vi "SetToRandomPosition.vi"(8 "error in (no error)":errorcluster, 10 "BlockedSpots":T1[](array[typedef]), 11 "SnakeSwitch in":refnum<class "SnakeSwitch.lvclass">) -> (0 "error out":errorcluster, 3 "SnakeSwitch out":refnum<class "SnakeSwitch.lvclass">)   [LabVIEW 2019, in "RT_Game.lvlib" / "SnakeSwitch.lvclass"]
uses:
  SnakeSwitch.lvclass
  C:/Users/FreshBob/Dropbox/VIs/myRIO_GameConsole/RT/RT_Game/GameObject/GameObject.lvclass
  Game/Coordinate.ctl
  GameObject/GameObject.lvclass/GameObject.ctl
  GameObject/Write position.vi
  Game/Game.lvclass
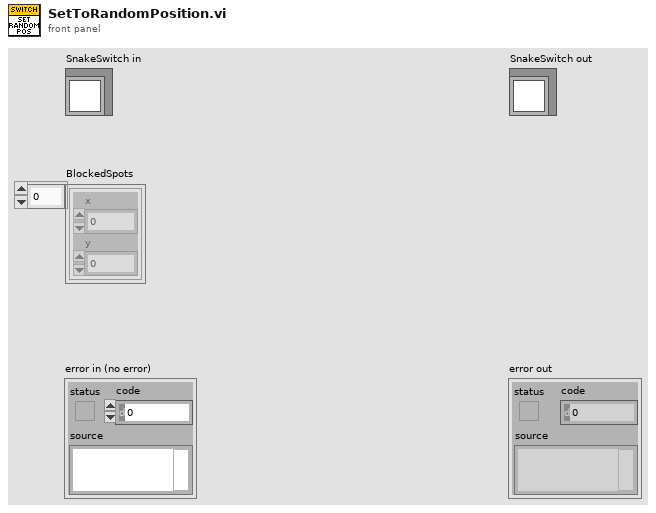
[diagram p1: front panel]
types:
  T1 = typedef "RT_Game.lvlib/Game.lvclass/Coordinate.ctl" = cluster{"x":dbl, "y":dbl}
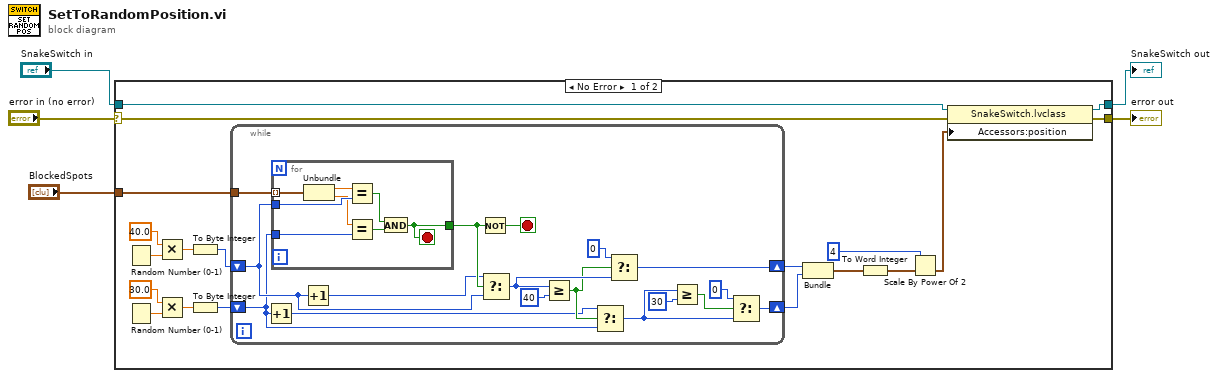
[diagram p0: block diagram]
diagram:
  n1 = case shown="No Error" "error in (no error)" {
    selector: "error in (no error)" -> [w24 w51]
    tunnel: [w14 w51] -> w4
    tunnel: [w12 w50] -> w2
    tunnel: "SnakeSwitch in" -> [w13 w50]
    tunnel: "BlockedSpots" -> [w15 _]
    frame No Error {
      n2 = Random Number (0-1)() -> (number: 0 to 1=w16:dbl)
      n3 = Random Number (0-1)() -> (number: 0 to 1=w20:dbl)
      n4 = Multiply(x=40.0, y=w16) -> (x*y=w18:dbl)
      n5 = Multiply(x=30.0, y=w20) -> (x*y=w21:dbl)
      n6 = To Byte Integer(number=w18) -> (8bit integer=w22:i8)
      n7 = To Byte Integer(number=w21) -> (8bit integer=w23:i8)
      n8 = while {
        shift-right: [w34] -> w11
        shift-left: w22 -> [w38]
        shift-right: [w27] -> w10
        shift-left: w23 -> [w31]
        tunnel: w15 -> [w41]
        stop <- w39 stop-if-true
        n9 = Increment(x=w31) -> (x+1=w30:i8)
        n10 = for {
          tunnel: w41 -> [w42] mode=indexing
          tunnel: w38 -> [w49]
          tunnel: w31 -> [w48]
          tunnel: [w45] -> w40
          stop <- w45 stop-if-true
          n11 = Unbundle(w42) -> ("x"=w44:dbl, "y"=w43:dbl)
          n12 = Equal?(x=w44, y=w49) -> (x = y?=w46:bool)
          n13 = Equal?(x=w43, y=w48) -> (x = y?=w47:bool)
          n14 = And(x=w46, y=w47) -> (x .and. y?=w45:bool)
        }
        n15 = Increment(x=w38) -> (x+1=w37:i8)
        n16 = Not(x=w40) -> (.not. x?=w39:bool)
        n17 = Select(t=w37, s=w40, f=w38) -> (s? t:f=w36:i8)
        n18 = Greater Or Equal?(x=w36, y=i8 40 ("x")) -> (x >= y?=w32:bool)
        n19 = Select(t=w30, s=w32, f=w31) -> (s? t:f=w29:i8)
        n20 = Select(t=i8 0, s=w32, f=w36) -> (s? t:f=w34:i8)
        n21 = Greater Or Equal?(x=w29, y=i8 30) -> (x >= y?=w26:bool)
        n22 = Select(t=i8 0, s=w26, f=w29) -> (s? t:f=w27:i8)
      }
      n23 = Bundle(w11, w10) -> (w9:cluster{i8, i8})  [unwired: 1 in]
      n24 = To Word Integer(number=w9) -> (16bit integer=w6:cluster{i16, i16})
      n25 = Scale By Power Of 2(n=i16 4, x=w6) -> (x*2^n=w8:cluster{i16, i16})
      n26 = property class="SnakeSwitch.lvclass"(reference=w13, error in=w24, "Accessors:position"=w8) -> (reference out=w12:refnum<class "SnakeSwitch.lvclass">, error out=w14:errorcluster)
    }
    frame Error {
    }
  }
  "error out" <- w4
  "SnakeSwitch out" <- w2
